vi "MakeExample.vi"(8 "error in (no error)":errorcluster, 9 "TriggerRefractoryPeriod (Frames)":i32, 10 "StimulusObject Parameters":variant, 11 "ConstantImageStimulus in":refnum<class "ConstantImageStimulus.lvclass">) -> (0 "error out":errorcluster, 3 "ConstantImageStimulus out":refnum<class "ConstantImageStimulus.lvclass">)   [LabVIEW 2019, in "ConstantImageStimulus.lvclass"]
uses:
  ConstantImageStimulus.lvclass
  <vilib>/vision/Image Controls.llb/IMAQ Image.ctl
  ConstantImageStimulus.lvclass/ConstantImageStimulus.ctl
  StimulusObject.lvclass
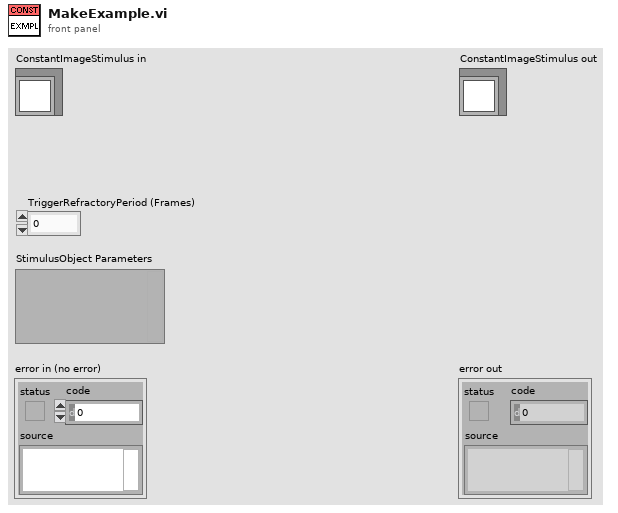
[diagram p1: front panel]
types:
  T1 = typedef "IMAQ Image.ctl" = refnum<image>
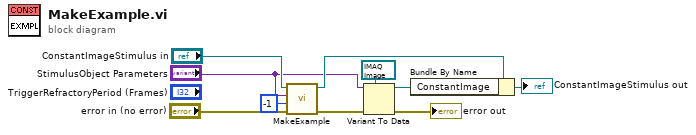
[diagram p0: block diagram]
diagram:
  n1 = call-parent "MakeExample.vi"("error in (no error)"="error in (no error)", "TriggerRefractoryPeriod (Frames)"=-1, "StimulusObject Parameters"="StimulusObject Parameters", "StimulusObject in"="ConstantImageStimulus in") -> ("error out"=w6:errorcluster, "StimulusObject out"=w8:refnum<class "ConstantImageStimulus.lvclass">)  [unwired: 6 in]
  n2 = Variant To Data(error in=w6, type=T1 refnum ("ConstantImage"), Variant="StimulusObject Parameters") -> (data=w3:T1, error out=→"error out":errorcluster)
  n3 = Bundle By Name(cluster=w8, "ConstantImage"=w3) -> (→"ConstantImageStimulus out":refnum<class "ConstantImageStimulus.lvclass">)
